vi "PrintHello.vi"(8 "error in (no error)":errorcluster, 11 "ProductB in":refnum<class "ProductB.lvclass">) -> (0 "error out":errorcluster, 3 "ProductB out":refnum<class "ProductB.lvclass">)   [LabVIEW 2016, in "ProductB.lvclass"]
uses:
  ProductA/ProductB.lvclass
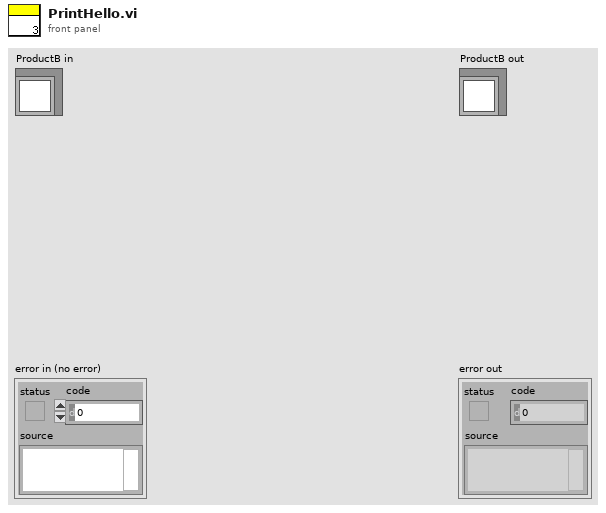
[diagram p1: front panel]
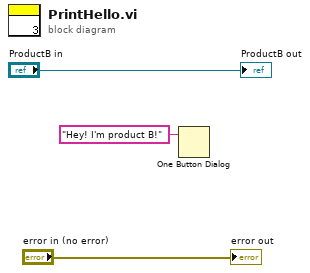
[diagram p0: block diagram]
diagram:
  n1 = One Button Dialog(message="Hey! I'm product B!") -> ()  [unwired: 1 in, 1 out]
  "error out" <- "error in (no error)"
  "ProductB out" <- "ProductB in"
